vi "Cycle Digital Output.vi"(0 "UI Power Line":tag, 2 "First Wait (sec)":dbl, 3 "Second Wait (sec)":dbl, 11 "Error In":errorcluster) -> (15 "Error Out":errorcluster)   [LabVIEW 2016]
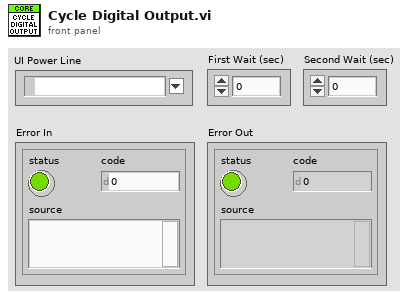
[diagram p1: front panel]
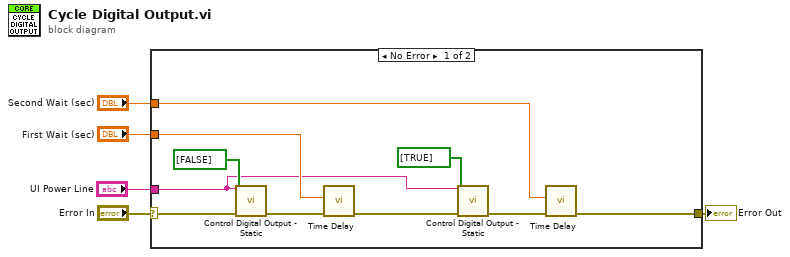
[diagram p0: block diagram]
diagram:
  n1 = case shown="No Error" "Error In" {
    selector: "Error In" -> [w9 w16]
    tunnel: "First Wait (sec)" -> [w13 _]
    tunnel: "UI Power Line" -> [w10 _]
    tunnel: [w6 w16] -> w3
    tunnel: "Second Wait (sec)" -> [w7 _]
    frame No Error {
      n2 = call "Control Digital Output - Static.vi"("Line(s)"=w10, "Output Array"=bool[] [FALSE], "Error In"=w9) -> ("Error Out"=w14:errorcluster)  [unwired: 12 in]
      n3 = call "Time Delay"("error in (no error)"=w14, "Delay Time (s)"=w13) -> ("error out"=w12:errorcluster)  [unwired: 9 in]
      n4 = call "Control Digital Output - Static.vi"("Line(s)"=w10, "Output Array"=bool[] [TRUE], "Error In"=w12) -> ("Error Out"=w8:errorcluster)  [unwired: 12 in]
      n5 = call "Time Delay"("error in (no error)"=w8, "Delay Time (s)"=w7) -> ("error out"=w6:errorcluster)  [unwired: 9 in]
    }
    frame Error {
    }
  }
  "Error Out" <- w3
